vi "MICSD Set Register.vi"(7 "Execute on Remote?(F)":bool, 8 "error in (no error)":errorcluster, 9 "Data":u8 format="%02x", 10 "Address":u16 format="%04x", 11 "VISA Resource Name":refnum<visa-resource-name>) -> (0 "error out":errorcluster, 3 "dup VISA Resource Name":refnum<visa-resource-name>)   [LabVIEW 2020]
uses:
  <vilib>/Instr/_visa.llb/VISA Configure Serial Port (Instr).vi
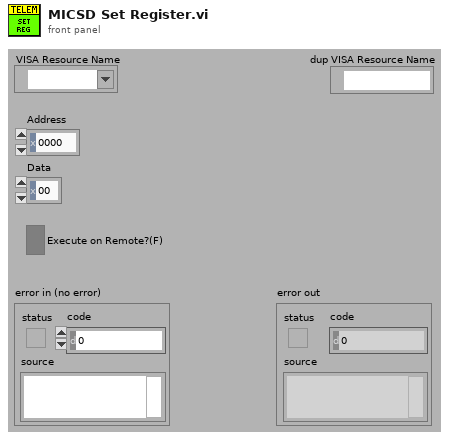
[diagram p1: front panel]
types:
  T1 = cluster{"Command Token":u8, "Length":u16, "Pack Data":u8[]}
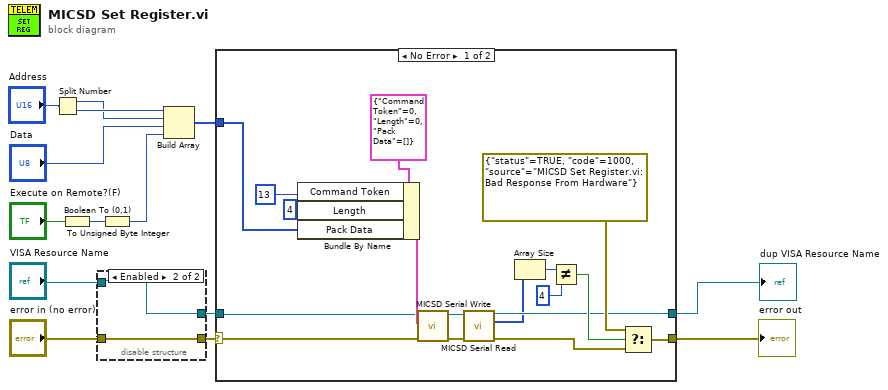
[diagram p0: block diagram]
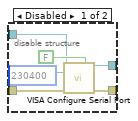
[diagram p2: hidden frame]
diagram:
  n1 = Split Number(x="Address") -> (hi(x)=w7:u8, lo(x)=w8:u8)
  n2 = Boolean To (0,1)(Boolean="Execute on Remote?(F)") -> (0, 1=w4:i16)
  n3 = disable-structure shown="Enabled" {
    disable-tunnel: [w18 w21] -> w13
    disable-tunnel: "error in (no error)" -> [w17 w21]
    disable-tunnel: "VISA Resource Name" -> [w16 w22]
    disable-tunnel: [w15 w22] -> w10
    frame Disabled {
      n4 = call-poly "VISA Configure Serial Port"("VISA resource name"=w16, "Enable Termination\nChar (T)"=FALSE ("Enable Termination\nChar (T)"), "baud rate (9600)"=u32 230400, "error in (no error)"=w17) -> ("VISA resource name out"=w15:refnum<visa-resource-name>, "error out"=w18:errorcluster)  [unwired: 10 in]
    }
    frame Enabled {
    }
  }
  n5 = To Unsigned Byte Integer(number=w4) -> (unsigned 8bit integer=w2:u8)
  n6 = Build Array(w8, w7, "Data", w2) -> (w1:u8[])
  n7 = case shown="No Error" w13 {
    selector: w13 -> [w37 w41]
    tunnel: [w24 w41] -> w9
    tunnel: w10 -> [w36 w40]
    tunnel: [w27 w40] -> w14
    tunnel: w1 -> [w23 _]
    frame No Error {
      n8 = Bundle By Name(cluster=T1 {"Command Token"=0, "Length"=0, "Pack Data"=[]} ("Write Data"), "Command Token"=u16 13 ("Length"), "Length"=u16 4, "Pack Data"=w23) -> (w39:T1)
      n9 = call "MICSD Serial Write.vi"("error in (no error)"=w37, "Write Data"=w39, "VISA Resource Name"=w36) -> ("error out"=w33:errorcluster, "DUP Visa Resource Name"=w34:refnum<visa-resource-name>)  [unwired: 7 in]
      n10 = call "MICSD Serial Read.vi"("error in (no error)"=w33, "VISA Resource Name"=w34) -> ("error out"=w25:errorcluster, "Read Data"=w26:u8[], "DUP Visa Resource Name"=w27:refnum<visa-resource-name>)  [unwired: 7 in]
      n11 = Array Size(array=w26) -> (size(s)=w30:i32)
      n12 = Not Equal?(x=w30, y=4) -> (x != y?=w29:bool)
      n13 = Select(t=errorcluster {"status"=TRUE, "code"=1000, "source"="MICSD Set Register.vi:  Bad Response From Hardware"} ("error IO"), s=w29, f=w25) -> (s? t:f=w24:errorcluster)
    }
    frame Error {
    }
  }
  "dup VISA Resource Name" <- w14
  "error out" <- w9
